vi "GFITS_ExecPostProc.vi"(6 "background":bool, 7 "args":string, 8 "error in (no error)":errorcluster, 9 "impath":string, 10 "postproc":string) -> (0 "error out":errorcluster, 2 "return type":i32)   [LabVIEW 2016]
uses:
  c/lib/libgfitspp.so
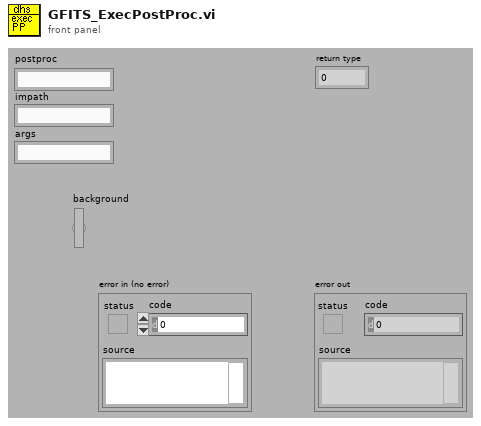
[diagram p1: front panel]
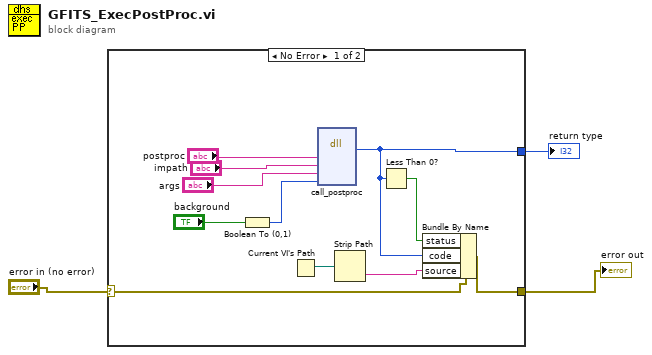
[diagram p0: block diagram]
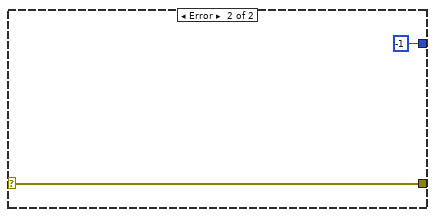
[diagram p2: hidden frame]
diagram:
  n1 = case shown="No Error" "error in (no error)" {
    selector: "error in (no error)" -> [w6 w16]
    tunnel: [w8 -1 ("return type")] -> w3
    tunnel: [w9 w16] -> w1
    frame No Error {
      n2 = Boolean To (0,1)(Boolean="background") -> (0, 1=w10:i16)
      n3 = Current VI's Path() -> (path=w5:path)
      n4 = dll-call lib="home/simager/panview/PAN/Modules/GFITS/private/c/lib/libgfitspp.so" fn="call_postproc"("ppath"="postproc", "impath"="impath", "args"="args", "back"=w10) -> ("return type"=w8:i32)  [unwired: 7 in, 2 out]
      n5 = Strip Path(path=w5) -> (name=w4:string)  [unwired: 1 out]
      n6 = Less Than 0?(x=w8) -> (x < 0?=w7:bool)
      n7 = Bundle By Name(cluster=w6, "status"=w7, "code"=w8, "source"=w4) -> (w9:errorcluster)
    }
    frame Error {
    }
  }
  "error out" <- w1
  "return type" <- w3
